vi "delete genealogy in folder.vi"(11 "Folder Path":path) -> (0 "error out":errorcluster)   [LabVIEW 2013]
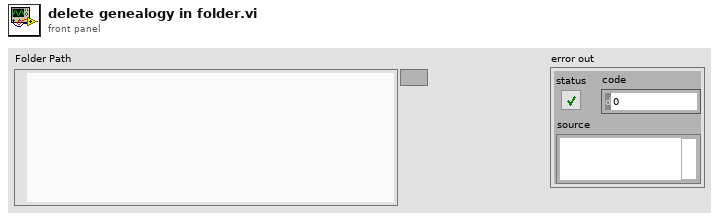
[diagram p1: front panel]
types:
  T1 = enum16{"open", "replace", "create", "open or create", "replace or create", "replace or create with confirmation"}
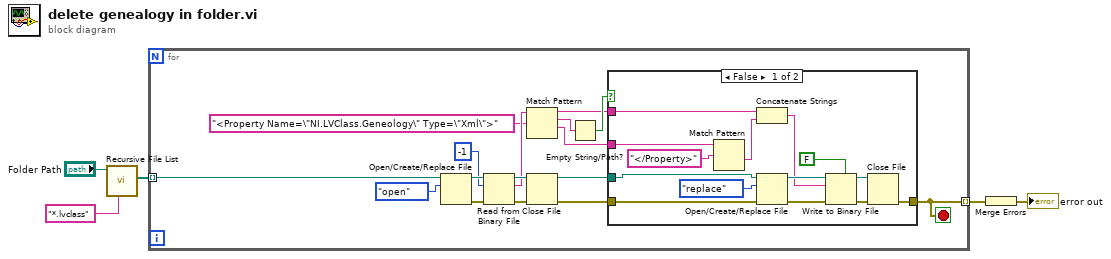
[diagram p0: block diagram]
diagram:
  n1 = call <vilib>:"Recursive File List.vi"("pattern"="*.lvclass", "Folder Path"="Folder Path") -> ("All Files in Dir"=w1:path[])  [unwired: 5 in, 4 out]
  n2 = for {
    tunnel: [w10] -> w5 mode=indexing
    tunnel: w1 -> [w21] mode=indexing
    stop <- w10 stop-if-true
    n3 = Open/Create/Replace File(file path (use dialog)=w21, operation (0:open)=T1."open") -> (refnum out=w19:refnum<file>, error out=w18:errorcluster)  [unwired: 4 in, 1 out]
    n4 = Read from Binary File(8:w18, 10:-1 ("count (1)"), 11:w19) -> (0:w15:errorcluster, 2:w14:string, 3:w16:refnum<file>)  [unwired: 3 in, 1 out]
    n5 = Match Pattern(string=w14, regular expression="<Property Name=\"NI.LVClass.Geneology\" Type=\"Xml\">") -> (before substring=w8:string, match substring=w12:string, after substring=w7:string)  [unwired: 1 in, 1 out]
    n6 = Close File(refnum=w16, error in=w15) -> (path=w6:path, error out=w9:errorcluster)
    n7 = Empty String/Path?(string/path=w12) -> (empty?=w11:bool)
    n8 = case shown="False" w11 {
      tunnel: [w24 w36] -> w10
      tunnel: w9 -> [w30 w36]
      tunnel: w8 -> [w33 _]
      tunnel: w7 -> [w35 _]
      tunnel: w6 -> [w29 _]
      frame False {
        n9 = Match Pattern(string=w35, regular expression="</Property>") -> (after substring=w32:string)  [unwired: 1 in, 3 out]
        n10 = Concatenate Strings(w33, w32) -> (w23:string)
        n11 = Open/Create/Replace File(file path (use dialog)=w29, error in=w30, operation (0:open)=T1."replace") -> (refnum out=w28:refnum<file>, error out=w27:errorcluster)  [unwired: 3 in, 1 out]
        n12 = Write to Binary File(file (use dialog)=w28, data=w23, error in=w27, 5:FALSE ("prepend array or string size? (T)")) -> (refnum out=w25:refnum<file>, error out=w26:errorcluster)  [unwired: 2 in, 1 out]
        n13 = Close File(refnum=w25, error in=w26) -> (error out=w24:errorcluster)  [unwired: 1 out]
      }
      frame True {
      }
    }
  }
  n14 = Merge Errors(w5) -> (→"error out":errorcluster)
